vi "niRFUtil FTW Generate Synchronously Tuned IIR Filter.vi"(1 "Poles (5)":i32=5, 2 "Sampling Period (sec)":dbl format="%^.2e", 3 "RBW (Hz)":dbl format="%^.2e") -> (0 "Filter":T1 {"Group Delay (sec)" format="%^.2e"; "Filter"."Forward Coefficients" format="%.4f"; "Filter"."Reverse Coefficients" format="%.4f"})   [LabVIEW 2015, in "niRFUtil.lvlib"]
doc: "(c) Copyright 2006, National Instruments, Inc. This VI may not be duplicated, sold, or distributed without written consent from National Instruments."
uses:
  niRFUtil.lvlib
  Includes/niRFUtil INC IIR Filter.ctl
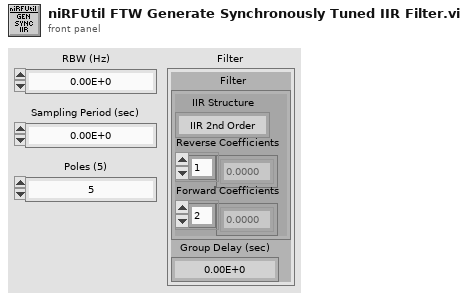
[diagram p1: front panel]
types:
  T1 = typedef "niRFUtil.lvlib/niRFUtil INC IIR Filter.ctl" = cluster{"Filter":cluster{"IIR Structure":enum32{"IIR 2nd Order", "IIR 4th Order"}, "Reverse Coefficients":dbl[], "Forward Coefficients":dbl[]}, "Group Delay (sec)":dbl}
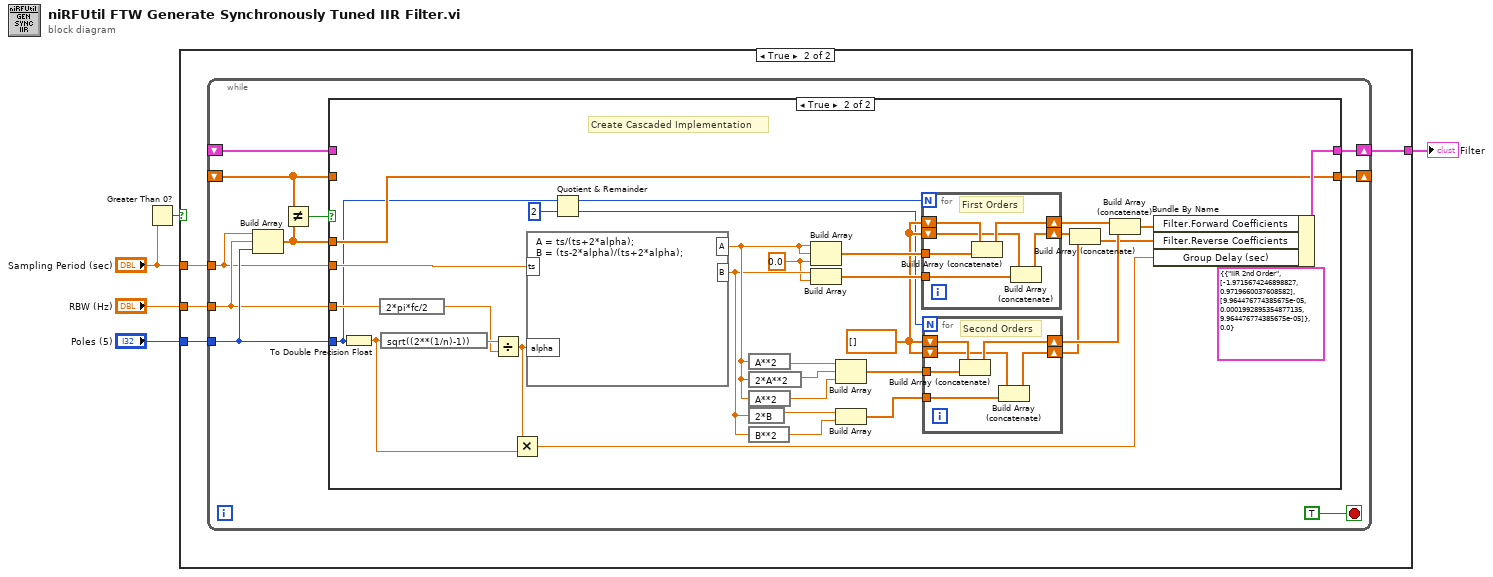
[diagram p0: block diagram]
diagram:
  n1 = Greater Than 0?(x="Sampling Period (sec)") -> (x > 0?=w1:bool)
  n2 = case shown="True" w1 {
    tunnel: "RBW (Hz)" -> [_ w9]
    tunnel: "Sampling Period (sec)" -> [_ w8]
    tunnel: [_ w7] -> w4
    tunnel: "Poles (5)" -> [_ w6]
    frame False {
    }
    frame True {
      n3 = while {
        shift-right: [w19] -> w7
        shift-left: _ -> [w18]
        shift-right: [w17] -> _
        shift-left: _ -> [w15]
        tunnel: w8 -> [w12]
        tunnel: w9 -> [w13]
        tunnel: w6 -> [w14]
        stop <- TRUE stop-if-true
        n4 = Build Array(w12, w13, w14) -> (w16:dbl[])
        n5 = Not Equal?(x=w15, y=w16) -> (x != y?=w10:bool)
        n6 = case shown="True" w10 {
          tunnel: [w21 w53] -> w19
          tunnel: w18 -> [w21 _]
          tunnel: [w20 w52] -> w17
          tunnel: w16 -> [_ w52]
          tunnel: w15 -> [w20 _]
          tunnel: w14 -> [_ w34]
          tunnel: w13 -> [_ w51]
          tunnel: w12 -> [_ w48]
          frame False {
          }
          frame True {
            w37 = dbl[] []
            w40 = 0.0 ("element")
            # "Create Cascaded Implementation"
            n7 = To Double Precision Float(number=w34) -> (double precision float=w23:dbl)
            n8 = expression code="2*pi*fc/2"(w51) -> (w49:dbl)
            n9 = expression code="sqrt((2**(1/n)-1))"(w23) -> (w50:dbl)
            n10 = Divide(x=w50, y=w49) -> (x/y=w24:dbl)
            n11 = Multiply(x=w24, y=w23) -> (x*y=w22:dbl)
            n12 = formula code="A = ts/(ts+2*alpha);\nB = (ts-2*alpha)/(ts+2*alpha);"("alpha"=w24, "ts"=w48) -> ("A"=w42:dbl, "B"=w41:dbl)
            n13 = Quotient & Remainder(x=w34, y=2) -> (x-y*floor(x/y)=w32:i32, floor(x/y)=w31:i32)
            n14 = expression code="A**2"(w42) -> (w47:dbl)
            n15 = expression code="2*A**2"(w42) -> (w46:dbl)
            n16 = expression code="A**2"(w42) -> (w45:dbl)
            n17 = expression code="2*B"(w41) -> (w44:dbl)
            n18 = expression code="B**2"(w41) -> (w43:dbl)
            n19 = Build Array(w42, w42, w40) -> (w39:dbl[])
            n20 = Build Array(w41, w40) -> (w38:dbl[])
            n21 = Build Array(w47, w46, w45) -> (w36:dbl[])
            n22 = Build Array(w44, w43) -> (w35:dbl[])
            n23 = for {
              N: w32 -> [_]
              shift-right: [w58] -> w30
              shift-left: w37 -> [w59]
              shift-right: [w55] -> w27
              shift-left: w37 -> [w56]
              tunnel: w39 -> [w60]
              tunnel: w38 -> [w57]
              # "First Orders"
              n24 = Build Array (concatenate)(w59, w60) -> (w58:dbl[])
              n25 = Build Array (concatenate)(w56, w57) -> (w55:dbl[])
            }
            n26 = for {
              N: w31 -> [_]
              shift-right: [w64] -> w29
              shift-left: w37 -> [w65]
              shift-right: [w61] -> w26
              shift-left: w37 -> [w62]
              tunnel: w36 -> [w66]
              tunnel: w35 -> [w63]
              # "Second Orders"
              n27 = Build Array (concatenate)(w65, w66) -> (w64:dbl[])
              n28 = Build Array (concatenate)(w62, w63) -> (w61:dbl[])
            }
            n29 = Build Array (concatenate)(w27, w26) -> (w25:dbl[])
            n30 = Build Array (concatenate)(w30, w29) -> (w28:dbl[])
            n31 = Bundle By Name(cluster=T1 {"Filter"={"IIR Structure"=enum."IIR 2nd Order", "Reverse Coefficients"=[-1.9715674246898827, 0.9719660037608582], "Forward Coefficients"=[9.964476774385675e-05, 0.0001992895354877135, 9.964476774385675e-05]}, "Group Delay (sec)"=0.0} ("RBW Filter"), "Filter.Forward Coefficients"=w28, "Filter.Reverse Coefficients"=w25, "Group Delay (sec)"=w22) -> (w53:T1)
          }
        }
      }
    }
  }
  "Filter" <- w4
